vi "Decimal Number to String & Length.vi"(2 "Decimal Number":dbl, 4 "Decimal Places (1)":i32=1) -> (6 "String":string, 7 "String Length":i32)   [LabVIEW 2021, in "Strings.lvlib"]
doc: "Converts a decimal number to a string and returns the length of the string.\nIf the number is an integer, it does not show any decimal part."
uses:
  Strings.lvlib
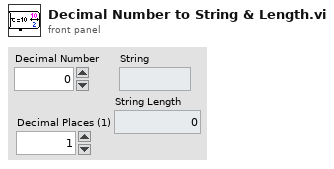
[diagram p1: front panel]
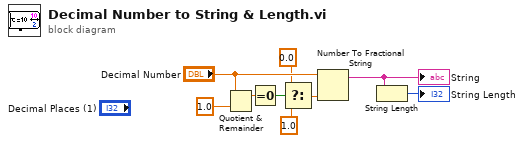
[diagram p0: block diagram]
diagram:
  n1 = Quotient & Remainder(x="Decimal Number", y=1.0) -> (x-y*floor(x/y)=w5:dbl)  [unwired: 1 out]
  n2 = Equal To 0?(x=w5) -> (x = 0?=w4:bool)
  n3 = Select(t=0.0, s=w4, f=1.0) -> (s? t:f=w3:dbl)
  n4 = Number To Fractional String(number="Decimal Number", precision (6)=w3) -> (F-format string=w9:string)  [unwired: 2 in]
  "String" <- w9
  n5 = String Length(string=w9) -> (length=→"String Length":i32)
